vi "I-SRC Configure (622X).vi"(5 "Voltage Limit":dbl min=-8.0 max=8.0, 7 "Current Level":dbl, 8 "error in (no error)":errorcluster, 11 "VISA resource name in":refnum<visa-resource-name>) -> (0 "error out":errorcluster, 3 "VISA resource name out":refnum<visa-resource-name>)   [LabVIEW 2016, in "Hall Effect Library.lvlib"]
uses:
  Hall Effect Library.lvlib
  <instrlib>/Keithley 622x/Keithley 622X.lvlib
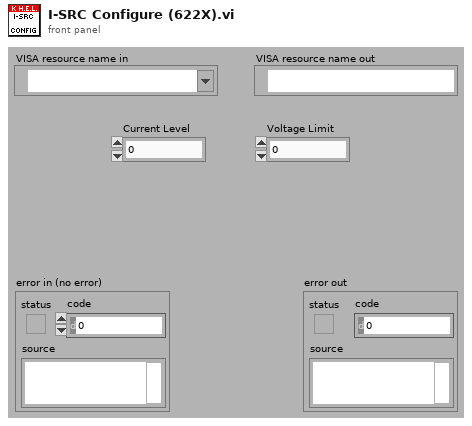
[diagram p1: front panel]
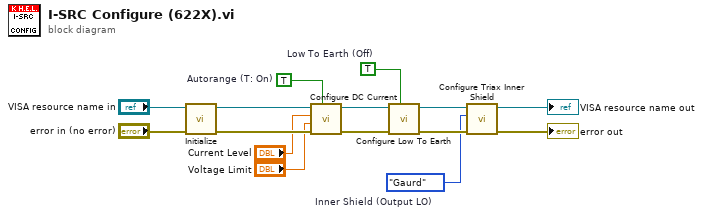
[diagram p0: block diagram]
diagram:
  w1 = enum16{"Output LO", "Gaurd"}."Gaurd"  # Inner Shield (Output LO)
  w2 = TRUE  # Low To Earth (Off)
  w13 = TRUE  # Autorange (T: On)
  n1 = call <instrlib>:"Initialize.vi"("error in (no error)"="error in (no error)", "VISA resource name"="VISA resource name in") -> ("error out"=w15:errorcluster, "VISA resource name out"=w14:refnum<visa-resource-name>)  [unwired: 3 in, 5 out]
  n2 = call <instrlib>:"Configure DC Current.vi"("Autorange (T: On)"=w13, "error in"=w15, "Compliance Level (10 V)"="Voltage Limit", "Current Level (0.0 A)"="Current Level", "VISA resource name"=w14) -> ("error out"=w8:errorcluster, "VISA resource name out"=w3:refnum<visa-resource-name>)  [unwired: 1 in, 4 out]
  n3 = call <instrlib>:"Configure Low To Earth.vi"("Low To Earth (Off)"=w2, "error in (no error)"=w8, "VISA resource name"=w3) -> ("error out"=w7:errorcluster, "VISA resource name out"=w4:refnum<visa-resource-name>)  [unwired: 7 out]
  n4 = call <instrlib>:"Configure Triax Inner Shield.vi"("error in (no error)"=w7, "Inner Shield (Output LO)"=w1, "VISA resource name"=w4) -> ("error out"=→"error out":errorcluster, "VISA resource name out"=→"VISA resource name out":refnum<visa-resource-name>)  [unwired: 7 out]
